vi "Sample in Container.vi"(6 "Queue timeout in ms (0)":i32, 7 "Action (Read)":enum16{"Read", "Publish"}(ring), 8 "error in (no error)":errorcluster, 9 "Read from SHV (F)":bool, 10 "Sample in":refnum<class "Sample.lvclass">, 11 "Sample Container":T1) -> (0 "error out":errorcluster, 1 "Queue timed out?":bool, 2 "Sample out":refnum<class "Sample.lvclass">, 3 "Sample Container":T1, 4 "Overflow Sample":refnum<class "Sample.lvclass">)   [LabVIEW 2015, in "cRIO-Carbondioxide.lvlib"]
uses:
  cRIO-Carbondioxide.lvlib
  Sample/Sample.lvclass
  Controls/Sample Container.ctl
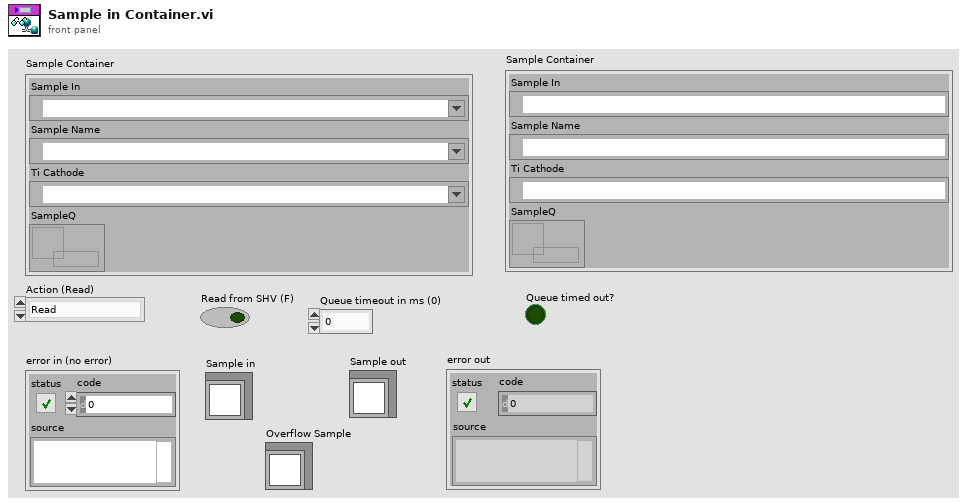
[diagram p1: front panel]
types:
  T1 = typedef "Sample Container.ctl" = cluster{"Sample In":refnum<k21>, "Sample Name":refnum<k21>, "Ti Cathode":refnum<k21>, "SampleQ":refnum<queue>}
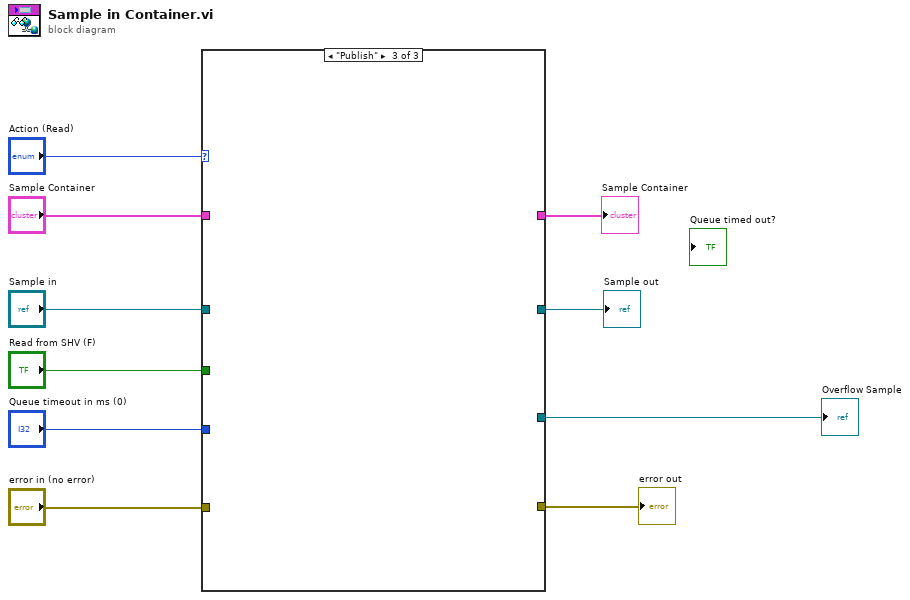
[diagram p0: block diagram]
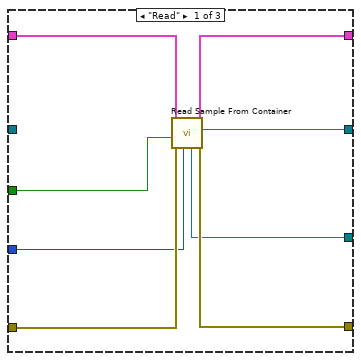
[diagram p2: hidden frame]
diagram:
  n1 = case shown="\"Publish\"" "Action (Read)" {
    tunnel: "error in (no error)" -> [w18 _ _]
    tunnel: "Sample Container" -> [w17 w20 _]
    tunnel: [w16 w20 _] -> w7
    tunnel: [w15 _ _] -> w6
    tunnel: "Read from SHV (F)" -> [w14 _ _]
    tunnel: "Queue timeout in ms (0)" -> [w13 _ _]
    tunnel: [w12 _ _] -> w3
    tunnel: [w11 w19 _] -> w2
    tunnel: "Sample in" -> [_ w19 _]
    frame "Read" {
      n2 = call "Read Sample From Container.vi"("Queue timeout in ms (-1)"=w13, "error in (no error)"=w18, "Read from SHV (F)"=w14, "Container"=w17) -> ("error out"=w15:errorcluster, "Sample out"=w11:refnum<class "Sample.lvclass">, "Container"=w16:T1, "Overflow Sample"=w12:refnum<class "Sample.lvclass">)  [unwired: 3 in, 1 out]
    }
    frame Default {
    }
    frame "Publish" {
    }
  }
  "error out" <- w6
  "Sample out" <- w2
  "Sample Container" <- w7
  "Overflow Sample" <- w3
